vi "Clear Cell Colors.vi"(0 "MulticolumnListbox in":refnum<vi>, 11 "error in (no error)":errorcluster) -> (4 "MulticolumnListbox out":refnum<vi>, 15 "error out":errorcluster)   [LabVIEW 2015, in "KTable.xctl"]
uses:
  KTable.xctl
  <vilib>/Utility/miscctls.llb/LVRowAndColumnTypeDef.ctl
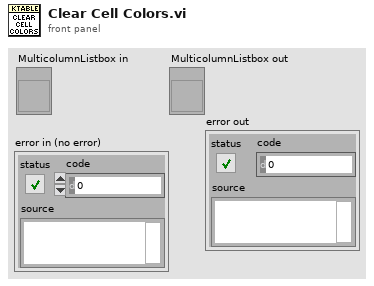
[diagram p1: front panel]
types:
  T1 = typedef "LVRowAndColumnTypeDef.ctl" = cluster{"Row":i32, "Column":i32}
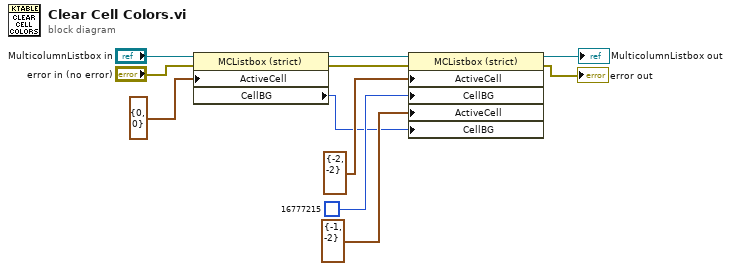
[diagram p0: block diagram]
diagram:
  n1 = property class="MCListbox (strict)"(reference="MulticolumnListbox in", error in="error in (no error)", "ActiveCell"=T1 {"Row"=0, "Column"=0} ("Active Cell:Active Cell")) -> (reference out=w9:refnum<vi>, error out=w8:errorcluster, "CellBG"=w2:u32)
  n2 = property class="MCListbox (strict)"(reference=w9, error in=w8, "ActiveCell"=T1 {"Row"=-2, "Column"=-2} ("Active Cell:Active Cell"), "CellBG"=u32 16777215, "ActiveCell"=T1 {"Row"=-1, "Column"=-2} ("Active Cell:Active Cell"), "CellBG"=w2) -> (reference out=→"MulticolumnListbox out":refnum<vi>, error out=→"error out":errorcluster)
